vi "gun_overide_data_store.vi"(10 "mode":enum16{"Set", "Get"}(ring), 11 "Overide":dbl) -> (3 "Overide Out":dbl)   [LabVIEW 2011]
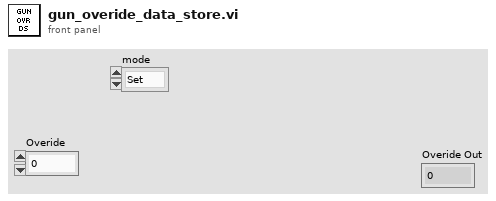
[diagram p1: front panel]
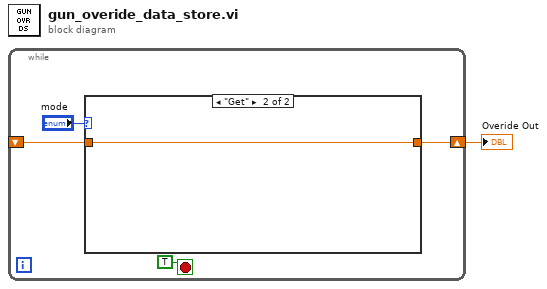
[diagram p0: block diagram]
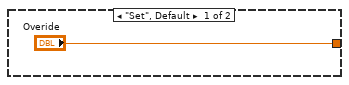
[diagram p2: hidden frame]
diagram:
  n1 = while {
    shift-right: [w3] -> w1
    shift-left: _ -> [w2]
    stop <- TRUE stop-if-true
    n2 = case shown="\"Get\"" "mode" {
      tunnel: ["Overide" w7] -> w3
      tunnel: w2 -> [_ w7]
      frame "Set", Default {
      }
      frame "Get" {
      }
    }
  }
  "Overide Out" <- w1
